vi "TCam_Focus.vi"(0 "Session in":T1, 1 "Focus <":bool, 2 "Autofocus":bool, 3 "Focus >":bool, 4 "Scale":u32=13, 5 "error in (no error)":errorcluster) -> (14 "Session Out":T1, 15 "FocusPos":u32, 19 "error out":errorcluster)   [LabVIEW 2024]
uses:
  <vilib>/userDefined/High Color/IMAQdx.ctl
  <resource>/objmgr/imaqdx.rc
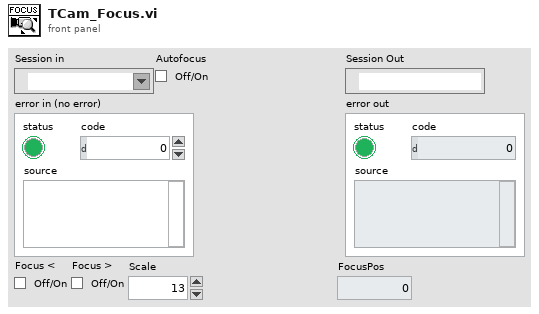
[diagram p1: front panel]
types:
  T1 = typedef "IMAQdx.ctl" = refnum<k21>
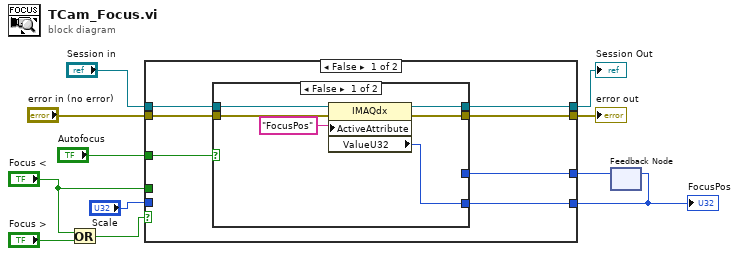
[diagram p0: block diagram]
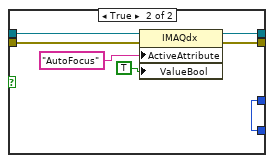
[diagram p2: hidden frame]
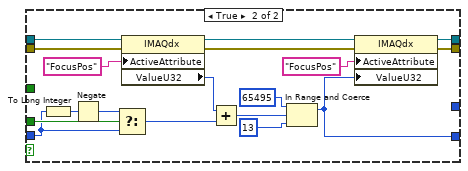
[diagram p3: hidden frame]
diagram:
  n1 = Or(x="Focus <", y="Focus >") -> (x .or. y?=w7:bool)
  n2 = feedback #1() -> (w2:u32)  [unwired: 1 in]
  n3 = case shown="False" w7 {
    tunnel: [w16 w49] -> w11
    tunnel: [w15 w48] -> w10
    tunnel: "Session in" -> [w18 w47]
    tunnel: "error in (no error)" -> [w17 w46]
    tunnel: "Focus <" -> [_ w36]
    tunnel: "Scale" -> [_ w34]
    tunnel: "Autofocus" -> [w14 _]
    tunnel: [w13 w32] -> w1
    tunnel: w2 -> [w12 _]
    frame False {
      n4 = case shown="False" w14 {
        tunnel: w18 -> [w23 w30]
        tunnel: w17 -> [w22 w28]
        tunnel: [w20 w27] -> w16
        tunnel: [w21 w26] -> w15
        tunnel: [w19 w25] -> w13
        tunnel: w12 -> [_ w25]
        frame False {
          n5 = property class="IMAQdx"(reference=w23, error in=w22, "ActiveAttribute"="FocusPos") -> (reference out=w20:T1, error out=w21:errorcluster, "ValueU32"=w19:u32)
        }
        frame True {
          n6 = property class="IMAQdx"(reference=w30, error in=w28, "ActiveAttribute"="AutoFocus", "ValueBool"=TRUE) -> (reference out=w27:T1, error out=w26:errorcluster)
        }
      }
    }
    frame True {
      n7 = To Long Integer(number=w34) -> (32bit integer=w33:i32)
      n8 = Negate(x=w33) -> (-x=w35:i32)
      n9 = Select(t=w35, s=w36, f=w34) -> (s? t:f=w37:u32)
      n10 = property class="IMAQdx"(reference=w47, error in=w46, "ActiveAttribute"="FocusPos") -> (reference out=w43:T1, error out=w42:errorcluster, "ValueU32"=w41:u32)
      n11 = Add(x=w41, y=w37) -> (x+y=w40:u32)
      n12 = In Range and Coerce(upper limit=u32 65495 ("lower limit"), x=w40, lower limit=u32 13) -> (coerced(x)=w32:u32)  [unwired: 1 out]
      n13 = property class="IMAQdx"(reference=w43, error in=w42, "ActiveAttribute"="FocusPos", "ValueU32"=w32) -> (reference out=w49:T1, error out=w48:errorcluster)
    }
  }
  "Session Out" <- w11
  "error out" <- w10
  "FocusPos" <- w1
  n14 = feedback-in #1(w1) -> ()
